vi "array to data claster.vi"(11 "Array":u64[](array[numeric])) -> (3 "Cluster":T1={"PW"=0, "frequency shift"=0.0, "amp"=0.9999923706054688, "mode type"=enum."CW", "mode depth"=0, "mode filter"=0, "phase shift"=0.0, "pulse shape filter"=0})   [LabVIEW 2021]
doc: "convert compresed data to PDW for the DDS"
uses:
  pulse_tx_vis/pdw.ctl
  pulse_tx_vis/CTL/mode_type.ctl
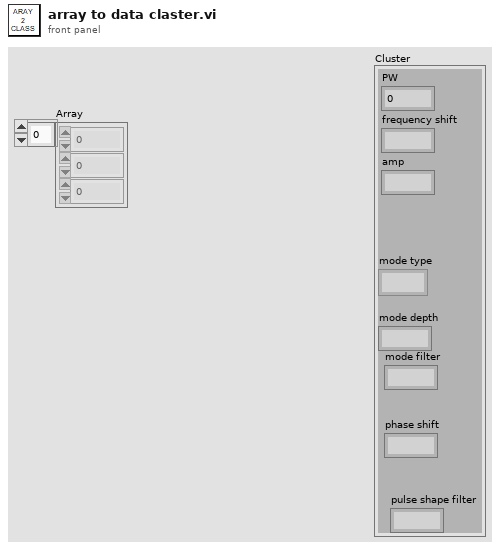
[diagram p1: front panel]
types:
  T1 = typedef "pdw.ctl" = cluster{"PW":u32, "frequency shift":fxp<+/-,48,0>, "amp":fxp<+/-,18,1>, "mode type":T2, "mode depth":u32, "mode filter":u8, "phase shift":fxp<+/-,16,1>, "pulse shape filter":u8}
  T2 = typedef "mode_type.ctl" = enum8{"CW", "NC - CW", "NC - cw", "LFM", "BPSK", "QPSK"}
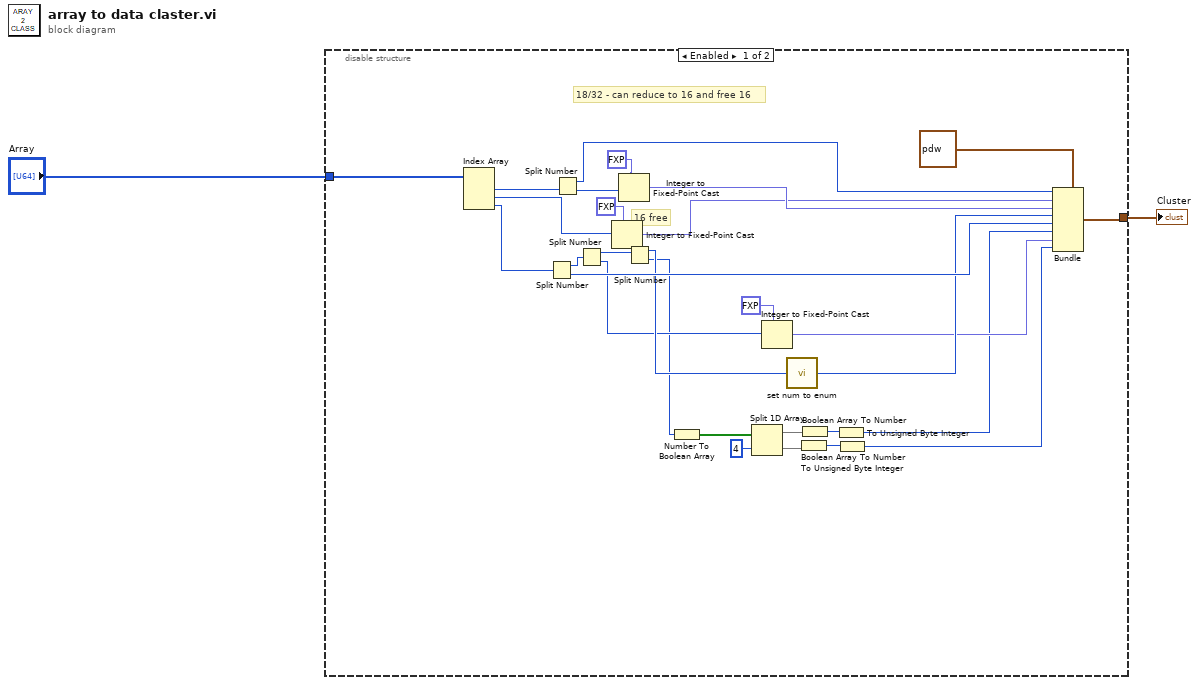
[diagram p0: block diagram]
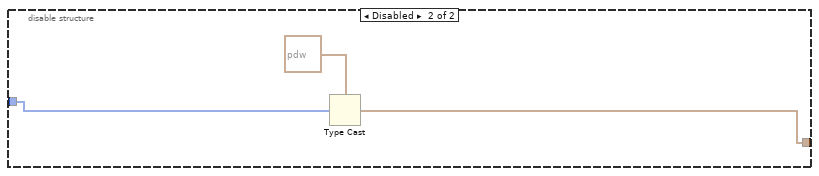
[diagram p2: hidden frame]
diagram:
  n1 = disable-structure shown="Enabled" {
    disable-tunnel: "Array" -> [w26 w33]
    disable-tunnel: [w24 w32] -> w1
    frame Enabled {
      # "16 free"
      # "18/32 - can reduce to 16 and free 16"
      n2 = Index Array(array=w26) -> (element #1=w27:u64, element #2=w29:u64, element #3=w20:u64)  [unwired: 3 in]
      n3 = Split Number(x=w20) -> (hi(x)=w18:u32, lo(x)=w19:u32)
      n4 = Split Number(x=w27) -> (hi(x)=w23:u32, lo(x)=w31:u32)
      n5 = Split Number(x=w18) -> (hi(x)=w17:u16, lo(x)=w12:u16)
      n6 = Integer to Fixed-Point Cast(fixed-point type=fxp<+/-,48,0> 0.0 ("frequency shift"), integer=w29) -> (fixed-point=w21:fxp<+/-,48,0>)
      n7 = Integer to Fixed-Point Cast(fixed-point type=fxp<+/-,18,1> 0.0 ("I"), integer=w31) -> (fixed-point=w22:fxp<+/-,18,1>)
      n8 = Split Number(x=w17) -> (hi(x)=w16:u8, lo(x)=w5:u8)
      n9 = Number To Boolean Array(number=w5) -> (Boolean array=w11:bool[])
      n10 = Split 1D Array(array=w11, index=4) -> (first subarray=w9:bool[], second subarray=w8:bool[])
      n11 = Integer to Fixed-Point Cast(fixed-point type=fxp<+/-,16,1> 0.0 ("phase shift"), integer=w12) -> (fixed-point=w13:fxp<+/-,16,1>)
      n12 = call "set num to enum.vi"("Numeric in"=w16) -> ("Numeric out"=w15:T2)
      n13 = Boolean Array To Number(Boolean array=w8) -> (number=w6:u32)
      n14 = Boolean Array To Number(Boolean array=w9) -> (number=w7:u32)
      n15 = To Unsigned Byte Integer(number=w7) -> (unsigned 8bit integer=w4:u8)
      n16 = To Unsigned Byte Integer(number=w6) -> (unsigned 8bit integer=w3:u8)
      n17 = Bundle(cluster=T1 {"PW"=0, "frequency shift"=0.0, "amp"=0.9999923706054688, "mode type"=enum."CW", "mode depth"=0, "mode filter"=0, "phase shift"=0.0, "pulse shape filter"=0} ("Cluster"), "PW"=w23, "frequency shift"=w21, "amp"=w22, "mode type"=w15, "mode depth"=w19, "mode filter"=w4, "phase shift"=w13, "pulse shape filter"=w3) -> (w24:T1)
    }
    frame Disabled {
      n18 = Type Cast(type=T1 {"PW"=0, "frequency shift"=0.0, "amp"=0.9999923706054688, "mode type"=enum."CW", "mode depth"=0, "mode filter"=0, "phase shift"=0.0, "pulse shape filter"=0} ("Cluster"), x=w33) -> (*(type *) &x=w32:T1)
    }
  }
  "Cluster" <- w1
